vi "Auton System Monitor.vi"(5 "Drive Motor Time (s)":dbl, 7 "Drive Motor Max Current":dbl, 10 "all currents (A)":dbl[](array[numeric]), 11 "Channels":i32[](array[numeric])) -> ()   [LabVIEW 2015]
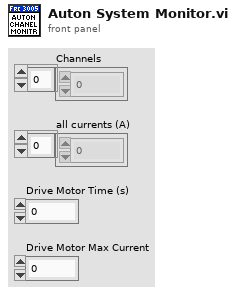
[diagram p1: front panel]
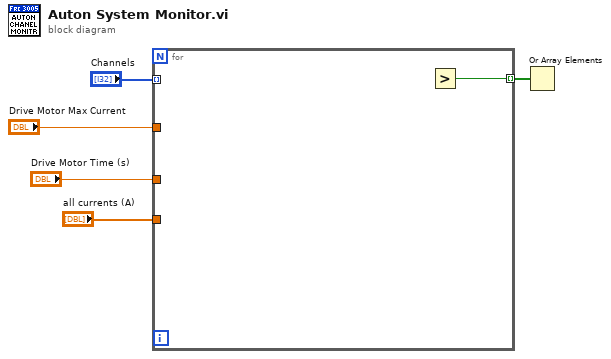
[diagram p0: block diagram]
diagram:
  n1 = for {
    tunnel: "all currents (A)" -> [_]
    tunnel: "Channels" -> [_] mode=indexing
    tunnel: [w6] -> w3 mode=indexing
    tunnel: "Drive Motor Time (s)" -> [_]
    tunnel: "Drive Motor Max Current" -> [_]
    n2 = Greater?() -> (0:w6:bool)  [unwired: 2 in]
  }
  n3 = Or Array Elements(Boolean array=w3) -> ()  [unwired: 1 out]
